vi "Write off1.vi"(8 "error in (no error)":errorcluster, 10 "off1":dbl[unit] min=-100.0 max=100.0, 11 "OffsetDef in":refnum<class "OffsetDef.lvclass">) -> (0 "error out":errorcluster, 3 "OffsetDef out":refnum<class "OffsetDef.lvclass">)   [LabVIEW 2014, in "TCSDataDefinitions.lvlib" / "TCSCommand.lvlib" / "OffsetCommands.lvlib" / "OffsetDef.lvclass"]
uses:
  OffsetDef.lvclass
  OffsetDef.lvclass/OffsetDef.ctl
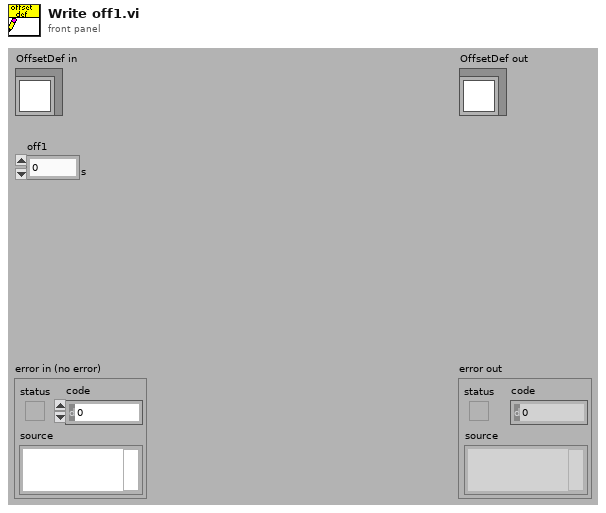
[diagram p1: front panel]
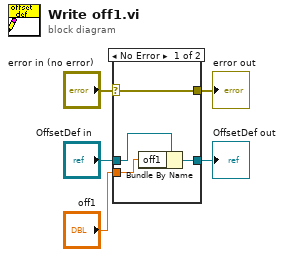
[diagram p0: block diagram]
diagram:
  n1 = case shown="No Error" "error in (no error)" {
    selector: "error in (no error)" -> [w9 w10]
    tunnel: [w9 w10] -> w4
    tunnel: [w7 w11] -> w2
    tunnel: "OffsetDef in" -> [w8 w11]
    tunnel: "off1" -> [w6 _]
    frame No Error {
      n2 = Bundle By Name(cluster=w8, "off1"=w6) -> (w7:refnum<class "OffsetDef.lvclass">)
    }
    frame Error {
    }
  }
  "error out" <- w4
  "OffsetDef out" <- w2
